vi "zmq_recv_event.vi"(4 "error in":errorcluster, 5 "timeout (none)":i32=-1, 6 "sockets":refnum<class "zmq_socket.lvclass">[](array[class]), 7 "poll event":refnum<user-event>) -> (0 "error out":errorcluster, 3 "poll event out":refnum<user-event>)   [LabVIEW 2020, in "zeromq.lvlib" / "zmq_socket.lvclass"]
doc: "Poll several sockets for input, and generate events when they receive data. This data can then be retrieved through an Event Structure.\n\nChecks whether each socket in <b>sockets</b> has data ready to receive, receives the data and raises an event. If no events happen within <b>timeout</b>, returns.\n\nIt is probably unsafe to use a <b>timeout</b> of 0, as if no data is received on any of the sockets, the LabVIEW process will hang indefinitely.\n\nMore details: http://sourceforge.net/p/labview-zmq/wiki/PollingAndEvents/"
uses:
  zmq_socket.lvclass
  poll_event_data.ctl
  socket_options.ctl
  poll_type.ctl
  zeromq.lvlib
panel:
  # "ØMQ"
  # "labview"
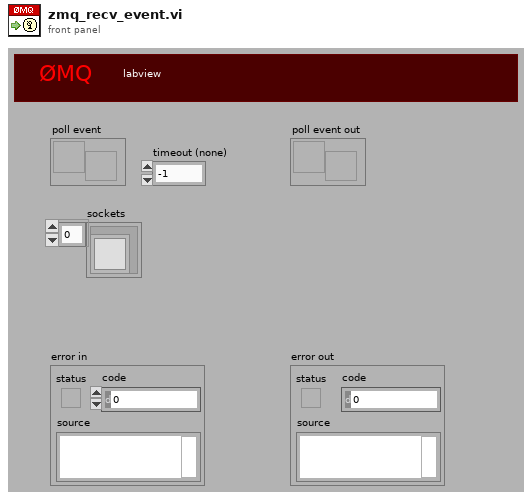
[diagram p1: front panel]
types:
  T1 = typedef "zeromq.lvlib/socket_options.ctl" = enum8{"NONE", "ZMQ_HWM", "<2>", "ZMQ_SWAP", "ZMQ_AFFINITY", "ZMQ_IDENTITY", "ZMQ_SUBSCRIBE", "ZMQ_UNSUBSCRIBE", "ZMQ_RATE", "ZMQ_RECOVERY_IVL", "ZMQ_MCAST_LOOP", "ZMQ_SNDBUF", "ZMQ_RCVBUF", "ZMQ_RCVMORE", "ZMQ_FD", "ZMQ_EVENTS", "ZMQ_TYPE", "ZMQ_LINGER", "ZMQ_RECONNECT_IVL", "ZMQ_BACKLOG", "ZMQ_RECOVERY_IVL_MSEC", "ZMQ_RECONNECT_IVL_MAX", "ZMQ_MAXMSGSIZE", "ZMQ_SNDHWM", "ZMQ_RCVHWM", "ZMQ_MULTICAST_HOPS", "<26>", "ZMQ_RCVTIMEO", "ZMQ_SNDTIMEO", "<29>", "<30>", "ZMQ_IPV4ONLY", "ZMQ_LAST_ENDPOINT", "ZMQ_ROUTER_MANDATORY", "ZMQ_TCP_KEEPALIVE", "ZMQ_TCP_KEEPALIVE_CNT", "ZMQ_TCP_KEEPALIVE_IDLE", "ZMQ_TCP_KEEPALIVE_INTVL", "ZMQ_TCP_ACCEPT_FILTER", "ZMQ_DELAY_ATTACH_ON_CONNECT", "ZMQ_XPUB_VERBOSE"}
  T2 = typedef "zeromq.lvlib/poll_type.ctl" = enum16{"None", "In", "Out", "In/Out"}
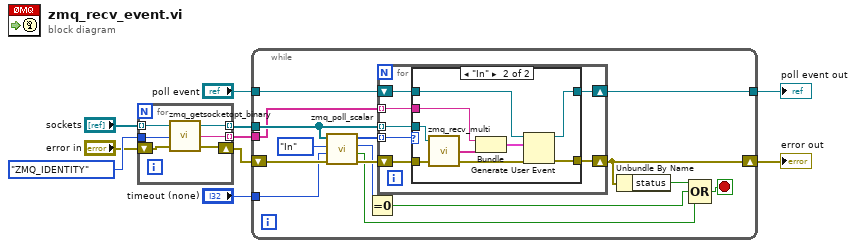
[diagram p0: block diagram]
diagram:
  n1 = for {
    tunnel: "sockets" -> [w16] mode=indexing
    tunnel: socket_options."ZMQ_IDENTITY" ("option") -> [w15]
    shift-right: [w13] -> w3
    shift-left: "error in" -> [w14]
    tunnel: [w12] -> w1 mode=indexing
    tunnel: [w11] -> w4 mode=indexing
    n2 = call "zmq_getsocketopt_binary.vi"("error in"=w14, "option"=w15, "socket in"=w16) -> ("error out"=w13:errorcluster, "value"=w12:string, "socket out"=w11:refnum<class "zmq_socket.lvclass">)
  }
  n3 = while {
    tunnel: w4 -> [w31]
    tunnel: "poll event" -> [w30]
    tunnel: [w29] -> w8
    shift-right: [w25] -> w10
    shift-left: w3 -> [w28]
    tunnel: "timeout (none)" -> [w19]
    tunnel: w1 -> [w17]
    stop <- w24 stop-if-true
    n4 = call "zmq_poll_scalar.vi"("error in"=w28, "timeout"=w19, "poll type"=poll_type."In", "sockets"=w31) -> ("error out"=w27:errorcluster, "timed out?"=w18:bool, "nevents"=w26:i32, "polled events"=w20:T2[])
    n5 = Equal To 0?(x=w26) -> (x = 0?=w23:bool)
    n6 = for {
      shift-right: [w37] -> w29
      shift-left: w30 -> [w38]
      shift-right: [w35] -> w25
      shift-left: w27 -> [w36]
      tunnel: w31 -> [w34] mode=indexing
      tunnel: w20 -> [w33] mode=indexing
      tunnel: w17 -> [w32] mode=indexing
      n7 = case shown="\"In\"" w33 {
        tunnel: w38 -> [w40 w49]
        tunnel: [w40 w48] -> w37
        tunnel: w36 -> [w39 w47]
        tunnel: [w39 w46] -> w35
        tunnel: w34 -> [_ w45]
        tunnel: w32 -> [_ w41]
        frame Default {
        }
        frame "In" {
          n8 = call "zmq_recv_multi.vi"("error in"=w47, "socket in"=w45) -> ("error out"=w42:errorcluster, "parts"=w43:string[])  [unwired: 1 in, 1 out]
          n9 = Bundle("value"=w41, "parts"=w43) -> (w44:cluster{"value":string, "parts":string[]})  [unwired: 1 in]
          n10 = Generate User Event(user event=w49, event data cluster=w44, error in=w42) -> (user event out=w48:refnum<user-event>, error out=w46:errorcluster)  [unwired: 1 in]
        }
      }
    }
    n11 = Unbundle By Name(w25) -> ("status"=w22:bool)
    n12 = Compound Arithmetic op=OR(w22, w23, w18) -> (w24:bool)
  }
  "error out" <- w10
  "poll event out" <- w8
